vi "Validate the Version.vi"(0 "Old Version":string[](array[string]), 5 "New Version":string[](array[string]), 11 "error in (no error)":errorcluster) -> (4 "Version Out":string[](array[string]), 15 "error out":errorcluster)   [LabVIEW 2021, in "Packager Helpers.lvlib"]
uses:
  Packager Helpers.lvlib
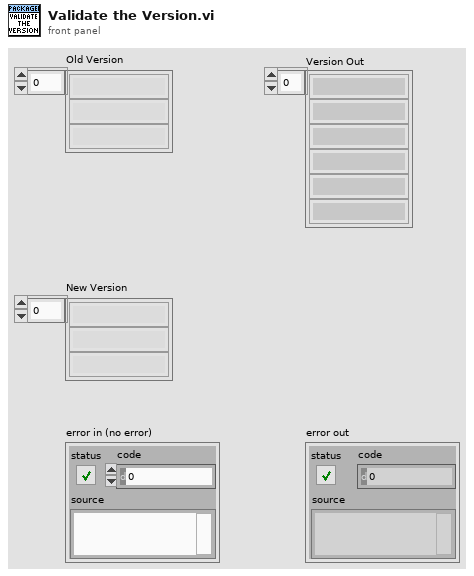
[diagram p1: front panel]
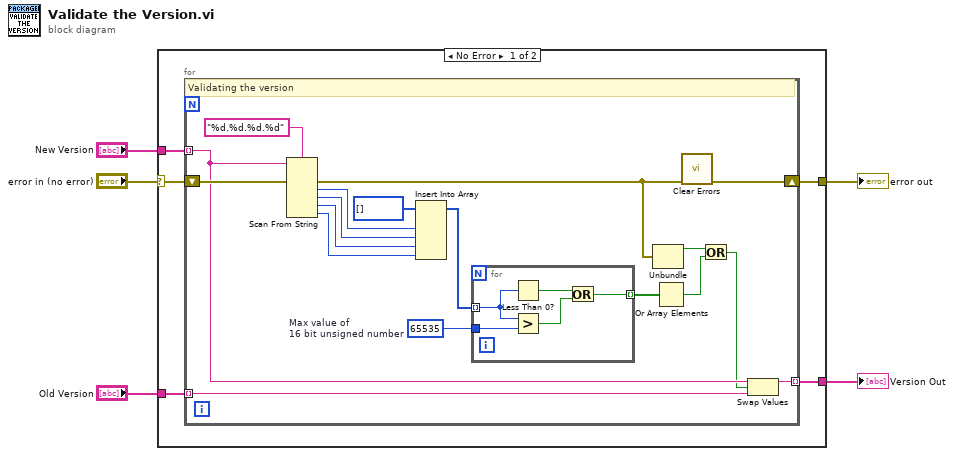
[diagram p0: block diagram]
diagram:
  n1 = case shown="No Error" "error in (no error)" {
    selector: "error in (no error)" -> [w6 w34]
    tunnel: "New Version" -> [w10 _]
    tunnel: [w8 w34] -> w3
    tunnel: [w7 _] -> w2
    tunnel: "Old Version" -> [w9 _]
    frame No Error {
      n2 = for {
        tunnel: w10 -> [w26] mode=indexing
        shift-right: [w14] -> w8
        shift-left: w6 -> [w28]
        tunnel: w9 -> [w16] mode=indexing
        tunnel: [w13] -> w7 mode=indexing
        w17 = 65535  # Max value of 16 bit unsigned number
        # "Validating the version"
        n3 = Scan From String(format string="%d.%d.%d.%d", input string=w26, error in=w28) -> (error out=w15:errorcluster, output 1=w25:i32, output 2=w24:i32, output 3=w23:i32, output 4=w22:i32)  [unwired: 5 in, 2 out]
        n4 = Insert Into Array(array=i32[] [], new element #1=w25, new element #2=w24, new element #3=w23, new element #4=w22) -> (w20:i32[])  [unwired: 1 in]
        n5 = for {
          tunnel: w20 -> [w29] mode=indexing
          tunnel: [w32] -> w19 mode=indexing
          tunnel: w17 -> [w31]
          n6 = Less Than 0?(x=w29) -> (x < 0?=w30:bool)
          n7 = Greater?(x=w29, y=w31) -> (0:w33:bool)
          n8 = Or(x=w30, y=w33) -> (x .or. y?=w32:bool)
        }
        n9 = Unbundle(w15) -> ("status"=w11:bool)  [unwired: 2 out]
        n10 = Or Array Elements(Boolean array=w19) -> (logical OR=w18:bool)
        n11 = call <vilib>:"Clear Errors.vi"("error in (no error)"=w15) -> ("error out"=w14:errorcluster)  [unwired: 5 in, 1 out]
        n12 = Or(x=w11, y=w18) -> (x .or. y?=w12:bool)
        n13 = Swap Values(12:w26, 13:w12, 14:w16) -> (1:w13:string)  [unwired: 1 out]
      }
    }
    frame Error {
    }
  }
  "error out" <- w3
  "Version Out" <- w2
